vi "4-bytes subarray to U32.vi"(9 "offset":i32, 11 "unsigned byte array":u8[](array[numeric])) -> (2 "U32 Out":u32, 3 "subarray out":u8[](array[numeric]))   [LabVIEW 2018, in "LV-0mq-Julia_roundtrip-lib.lvlib" / "LV2Julia_core.lvlib"]
uses:
  LV2Julia_core.lvlib
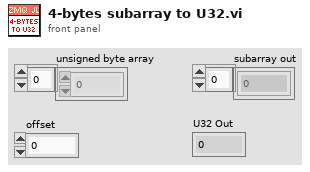
[diagram p1: front panel]
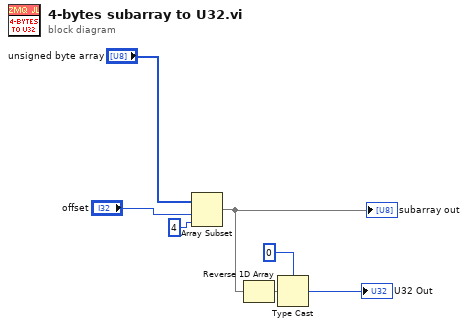
[diagram p0: block diagram]
diagram:
  n1 = Array Subset(array="unsigned byte array", index="offset", length=4) -> (w4:u8[])
  "subarray out" <- w4
  n2 = Reverse 1D Array(array=w4) -> (reversed array=w7:u8[])
  n3 = Type Cast(type=u32 0 ("length"), x=w7) -> (*(type *) &x=→"U32 Out":u32)
